vi "terminate.vi"(8 "error in (no error)":errorcluster, 11 "FPGA_AK101022Resonance in":refnum<class "FPGAWrapperAK101022Resonance.lvclass">) -> (0 "error out":errorcluster, 3 "FPGA_AK101022Resonance out":refnum<class "FPGAWrapperAK101022Resonance.lvclass">)   [LabVIEW 2010, in "FPGAWrapperAK101022Resonance.lvclass"]
uses:
  FPGAWrapperAK101022Resonance.lvclass
  GenericFPGAWrapper/GenericFPGAWrapper/GenericFPGAWrapper.lvclass
  class_data.vi
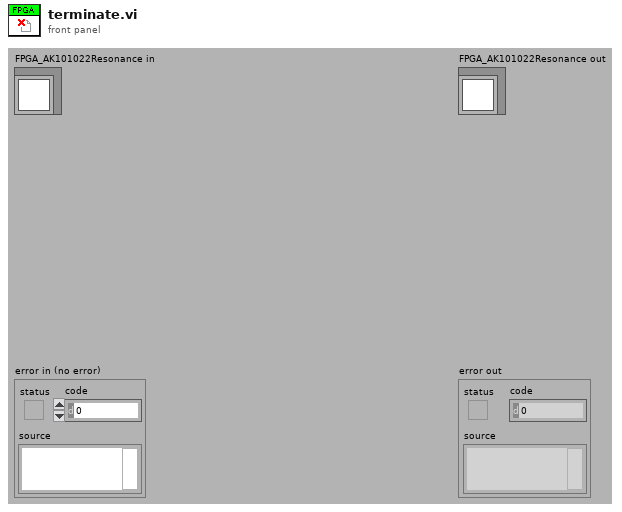
[diagram p1: front panel]
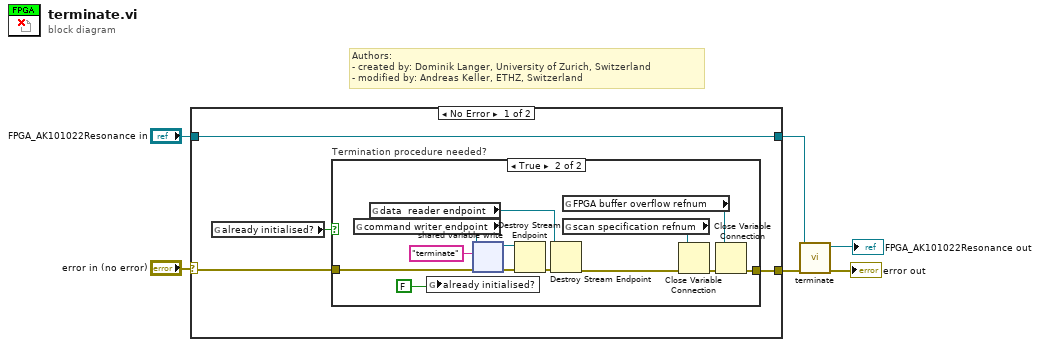
[diagram p0: block diagram]
diagram:
  # "Authors: \n- created by: Dominik Langer, University of Zurich, Switzerland\n- modified by: Andreas Keller, ETHZ, Switzerland"
  n1 = case shown="No Error" "error in (no error)" {
    selector: "error in (no error)" -> [w8 w26]
    tunnel: "FPGA_AK101022Resonance in" -> [w10 w25]
    tunnel: [w9 w26] -> w3
    tunnel: [w10 w25] -> w1
    frame No Error {
      n2 = global read "class_data.vi" "already initialised?"() -> (w7:bool)
      n3 = case "Termination procedure needed?" shown="True" w7 {
        tunnel: [w11 w13] -> w9
        tunnel: w8 -> [w11 w19]
        frame False {
        }
        frame True {
          n4 = global read "class_data.vi" "command writer endpoint"() -> (w24:refnum<k21>)
          n5 = global read "class_data.vi" "data  reader endpoint"() -> (w23:refnum<k21>)
          n6 = global write "class_data.vi" "already initialised?"(FALSE) -> ()
          n7 = shared-variable-write(w24, w19, "terminate" ("data in")) -> (w20:refnum<k21>, w22:errorcluster)  [unwired: 1 in, 1 out]
          n8 = Destroy Stream Endpoint(8:w22, 11:w20) -> (0:w21:errorcluster)
          n9 = Destroy Stream Endpoint(8:w21, 11:w23) -> (0:w14:errorcluster)
          n10 = global read "class_data.vi" "FPGA buffer overflow refnum"() -> (w16:refnum<k21>)
          n11 = global read "class_data.vi" "scan specification refnum"() -> (w12:refnum<k21>)
          n12 = Close Variable Connection(8:w14, 11:w12) -> (0:w15:errorcluster)
          n13 = Close Variable Connection(8:w15, 11:w16) -> (0:w13:errorcluster)
        }
      }
    }
    frame Error {
    }
  }
  n14 = call-parent "terminate.vi"("error in (no error)"=w3, "GenericPlugin in"=w1) -> ("error out"=→"error out":errorcluster, "GenericPlugin out"=→"FPGA_AK101022Resonance out":refnum<class "FPGAWrapperAK101022Resonance.lvclass">)  [unwired: 8 in]
